vi "Intensity Graph View Controller.vi"(0 "Intensity Graph":refnum<vi>, 5 "X":dbl[](array[numeric]), 7 "Y":dbl[](array[numeric]), 9 "Z":dbl[][](array[numeric]), 11 "error in (no error)":errorcluster) -> (4 "Intensity Graph Out":refnum<vi>, 15 "error out":errorcluster)   [LabVIEW 2016]
doc: "Use this template to build a VI to use as a subVI."
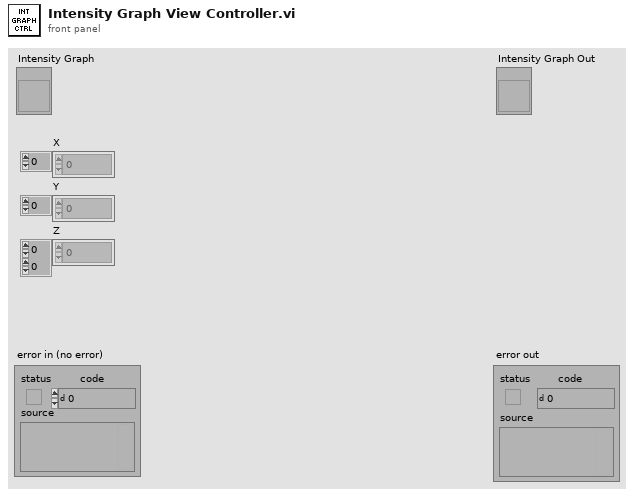
[diagram p1: front panel]
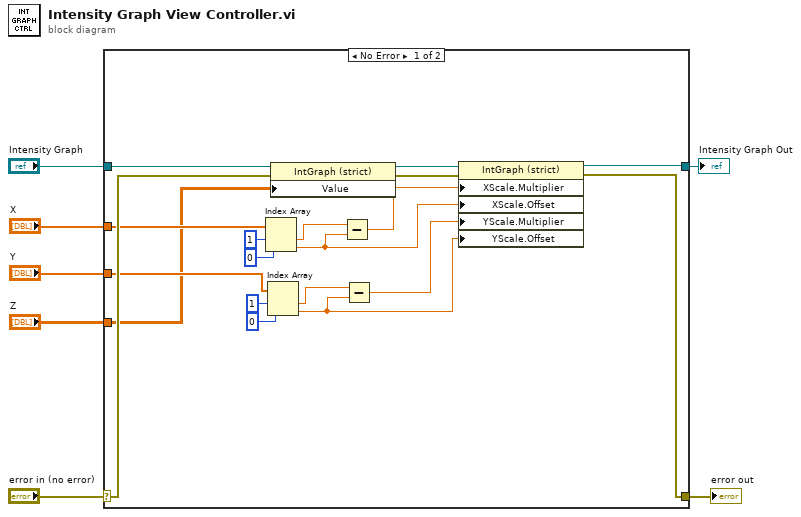
[diagram p0: block diagram]
diagram:
  n1 = case shown="No Error" "error in (no error)" {
    selector: "error in (no error)" -> [w13 w28]
    tunnel: [w12 w28] -> w6
    tunnel: "Intensity Graph" -> [w15 w27]
    tunnel: [w14 w27] -> w4
    tunnel: "X" -> [w10 _]
    tunnel: "Y" -> [w9 _]
    tunnel: "Z" -> [w8 _]
    frame No Error {
      n2 = Index Array(array=w10, index #1=1 ("index"), index #2=0 ("index")) -> (element #1=w23:dbl, element #2=w21:dbl)
      n3 = Index Array(array=w9, index #1=1 ("index"), index #2=0 ("index")) -> (element #1=w20:dbl, element #2=w16:dbl)
      n4 = property class="IntGraph (strict)"(reference=w15, error in=w13, "Value"=w8) -> (reference out=w26:refnum<vi>, error out=w11:errorcluster)
      n5 = Subtract(x=w23, y=w21) -> (x-y=w22:dbl)
      n6 = Subtract(x=w20, y=w16) -> (x-y=w17:dbl)
      n7 = property class="IntGraph (strict)"(reference=w26, error in=w11, "XScale.Multiplier"=w22, "XScale.Offset"=w21, "YScale.Multiplier"=w17, "YScale.Offset"=w16) -> (reference out=w14:refnum<vi>, error out=w12:errorcluster)
    }
    frame Error {
    }
  }
  "error out" <- w6
  "Intensity Graph Out" <- w4
